vi "Go to Coordinate.vi"() -> ()   [LabVIEW 2015]
panel:
  out "Finished?":bool
  in  "Distance Tolerances":dbl
  in  "Angle Tolerances":dbl
  in  "Position":cluster{"X":dbl, "Y":dbl, "Angle":dbl}
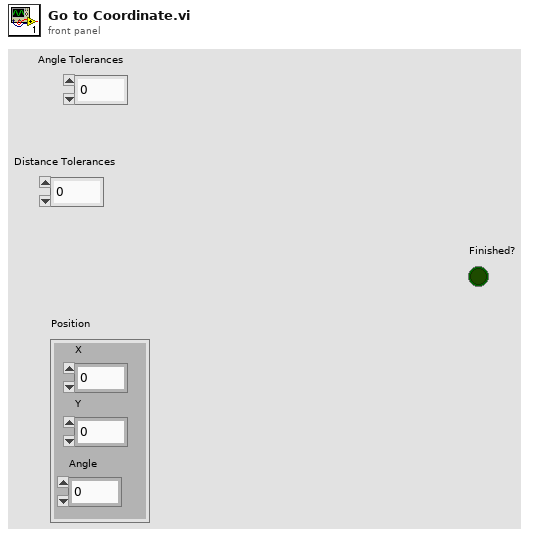
[diagram p1: front panel]
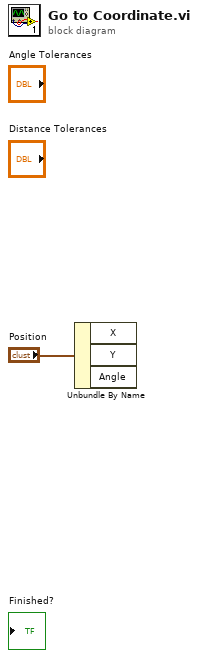
[diagram p0: block diagram]
diagram:
  n1 = Unbundle By Name("Position") -> ("Angle"=w1:dbl)  [unwired: 2 out]
